vi "SwitchState.vi"(6 "Switch Action":T1=enum."Initialize", 8 "error in (no error)":errorcluster, 9 "channel 2":string, 10 "channel 1":string, 11 "Switch Session":refnum<k15> caption="Switch Session In") -> (0 "error out":errorcluster, 2 "Switch State":string[](array[string]), 3 "Switch Session out":refnum<k15> caption="Switch Session Out")   [LabVIEW 2019, in "ctet_mux_User Library.lvlib"]
uses:
  ctet_mux_User Library.lvlib
  Types/Switch Action.ctl
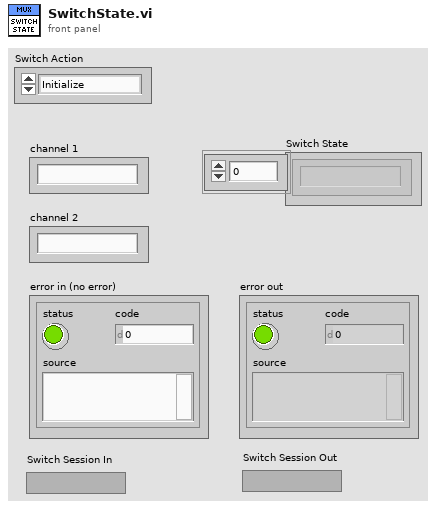
[diagram p1: front panel]
types:
  T1 = typedef "ctet_mux_User Library.lvlib/Switch Action.ctl" = enum16{"Get Switch State", "Initialize", "Connect Channel", "Disconnect Channel", "Close Relay", "Open Relay", "Disconnect/Open All"}
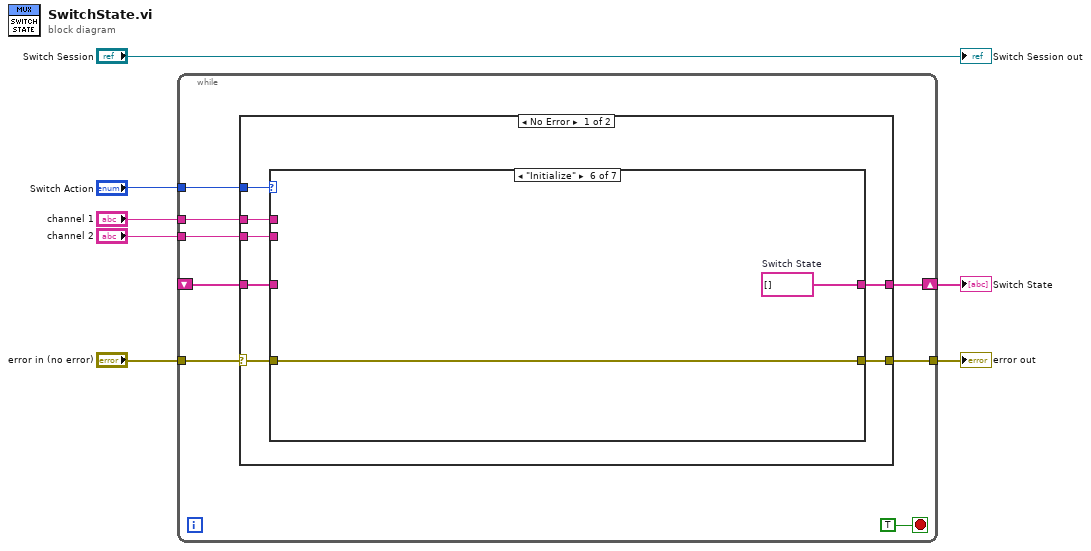
[diagram p0: block diagram]
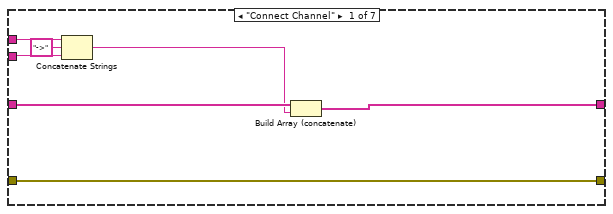
[diagram p2: hidden frame]
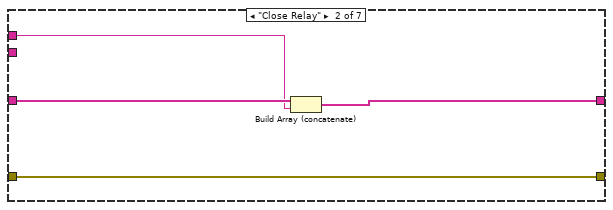
[diagram p3: hidden frame]
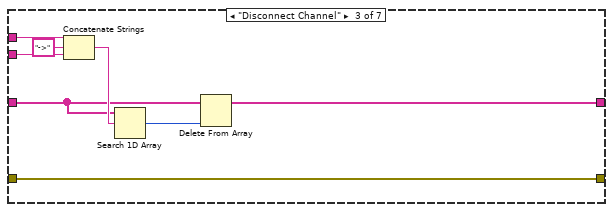
[diagram p4: hidden frame]
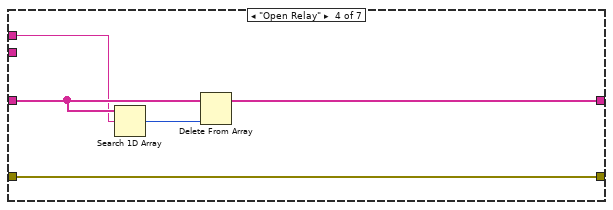
[diagram p5: hidden frame]
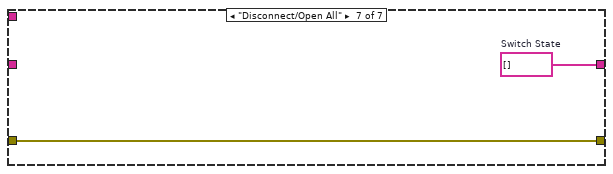
[diagram p7: hidden frame]
diagram:
  n1 = while {
    tunnel: "channel 1" -> [w13]
    tunnel: "channel 2" -> [w12]
    tunnel: "Switch Action" -> [w11]
    shift-right: [w10] -> w3
    shift-left: _ -> [w8]
    tunnel: "error in (no error)" -> [w14]
    tunnel: [w15] -> w7
    stop <- TRUE stop-if-true
    n2 = case shown="No Error" w14 {
      selector: w14 -> [w19 w53]
      tunnel: [w22 w53] -> w15
      tunnel: w13 -> [w21 _]
      tunnel: w12 -> [w20 _]
      tunnel: w11 -> [w18 _]
      tunnel: [w17 w54] -> w10
      tunnel: w8 -> [w16 w54]
      frame No Error {
        n3 = case shown="\"Initialize\"" w18 {
          tunnel: [w29 w33 w41 w46 w48 w50 w52] -> w22
          tunnel: w21 -> [w28 w30 w39 w42 _ _ _]
          tunnel: w20 -> [w26 _ w38 _ _ _ _]
          tunnel: w19 -> [w29 w33 w41 w46 w48 w50 w52]
          tunnel: [w23 w31 w34 w43 w47 w49 w51] -> w17
          tunnel: w16 -> [w25 w32 w36 w45 w47 _ _]
          frame "Connect Channel" {
            n4 = Concatenate Strings(w28, "->" ("string"), w26) -> (w24:string)
            n5 = Build Array (concatenate)(w25, w24) -> (w23:string[])
          }
          frame "Close Relay" {
            n6 = Build Array (concatenate)(w32, w30) -> (w31:string[])
          }
          frame "Disconnect Channel" {
            n7 = Concatenate Strings(w39, "->" ("string"), w38) -> (w37:string)
            n8 = Search 1D Array(1D array=w36, element=w37) -> (index of element=w35:i32)  [unwired: 1 in]
            n9 = Delete From Array(array=w36, index=w35) -> (array with subset deleted=w34:string[])  [unwired: 1 in, 1 out]
          }
          frame "Open Relay" {
            n10 = Search 1D Array(1D array=w45, element=w42) -> (index of element=w44:i32)  [unwired: 1 in]
            n11 = Delete From Array(array=w45, index=w44) -> (array with subset deleted=w43:string[])  [unwired: 1 in, 1 out]
          }
          frame "Get Switch State", Default {
          }
          frame "Initialize" {
            w49 = string[] []  # Switch State
          }
          frame "Disconnect/Open All" {
            w51 = string[] []  # Switch State
          }
        }
      }
      frame Error {
      }
    }
  }
  "error out" <- w7
  "Switch State" <- w3
  "Switch Session out" <- "Switch Session"
